vi "toggle.vi"(9 "Boolean 3":bool, 11 "Boolean":bool) -> (3 "Boolean 2":bool)   [LabVIEW 2019]
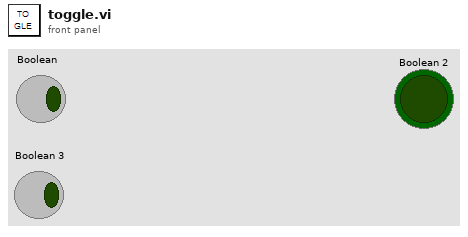
[diagram p1: front panel]
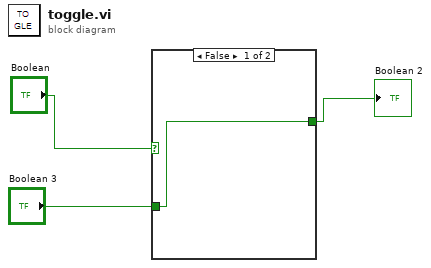
[diagram p0: block diagram]
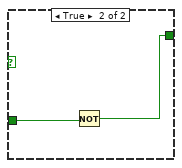
[diagram p2: hidden frame]
diagram:
  n1 = case shown="False" "Boolean" {
    tunnel: [w4 w5] -> w2
    tunnel: "Boolean 3" -> [w4 w6]
    frame False {
    }
    frame True {
      n2 = Not(x=w6) -> (.not. x?=w5:bool)
    }
  }
  "Boolean 2" <- w2
